vi "Array of I16_ASCII String To Data.vi"(8 "error in (no error)":errorcluster, 9 "Default":cluster{"I16 Array":i16[]}, 11 "Value":string) -> (0 "error out":errorcluster, 3 "Data":cluster{"I16 Array":i16[]})   [LabVIEW 2020, in "Current Value Table(Rebuild).lvlib"]
doc: "This VI converts data stored on disk as an ascii string into the correct data type. This VI must perform the opposite operation to the DataToASCIIString function."
uses:
  Current Value Table(Rebuild).lvlib
  Errors/Generate Error.vi
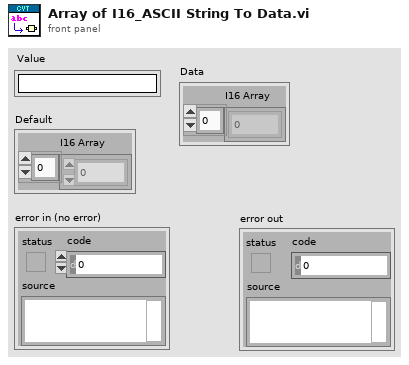
[diagram p1: front panel]
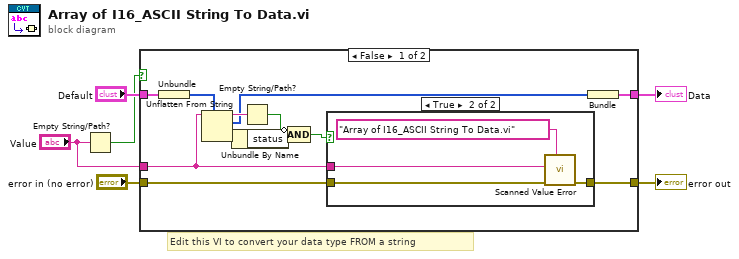
[diagram p0: block diagram]
diagram:
  # "Edit this VI to convert your data type FROM a string"
  n1 = Empty String/Path?(string/path="Value") -> (empty?=w3:bool)
  n2 = case shown="False" w3 {
    tunnel: "Default" -> [w16 w25]
    tunnel: "Value" -> [w8 _]
    tunnel: [w15 w25] -> w1
    tunnel: "error in (no error)" -> [w17 w24]
    tunnel: [w18 w24] -> w5
    frame False {
      n3 = Unbundle(w16) -> ("I16 Array"=w9:i16[])
      n4 = Unflatten From String(type=w9, binary string=w8) -> (rest of the binary string=w12:string, value=w10:i16[], error out=w11:errorcluster)  [unwired: 3 in]
      n5 = Unbundle By Name(w11) -> ("status"=w7:bool)
      n6 = Empty String/Path?(string/path=w12) -> (empty?=w14:bool)
      n7 = Compound Arithmetic op=AND(invert w14, w7) -> (w13:bool)
      n8 = case shown="True" w13 {
        tunnel: [w19 w23] -> w18
        tunnel: w17 -> [w19 w22]
        tunnel: w8 -> [_ w21]
        frame False {
        }
        frame True {
          n9 = call "Scanned Value Error.vi"("caller name"="Array of I16_ASCII String To Data.vi", "error in (no error)"=w22, "Value"=w21) -> ("error out"=w23:errorcluster)  [unwired: 8 in]
        }
      }
      n10 = Bundle("I16 Array"=w10) -> (w15:cluster{"I16 Array":i16[]})  [unwired: 1 in]
    }
    frame True {
    }
  }
  "error out" <- w5
  "Data" <- w1
